vi "PH_Interaction.Super Destroy Me.vi"(0 "i ref out":refnum<vi>) -> ()   [LabVIEW 2014, in "PH_Common.lvlib"]
doc: "This VI forces the super proc asks the super proc to desgtroy the referenced instance."
uses:
  CS_Core/CSSystem/CoreLib/CoreLib.string 2 byte array.vi
  PH_Common.lvlib
  CS_Core/BaseProcess/BaseProcess.lvlib
  CS_Core/CSSystem/CSSystemLib/CSSystemLib.lvlib
  CS_Core/CSSystem/CoreLib/CoreLib.lvlib
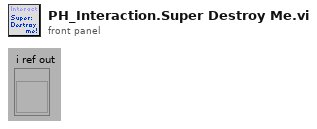
[diagram p1: front panel]
types:
  T1 = typedef "CoreDefs.rawDataType.ctl" = i8[]
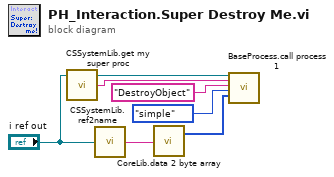
[diagram p0: block diagram]
diagram:
  n1 = call "CSSystemLib.get my super proc.vi"() -> ("name"=w2:string)  [unwired: 1 in]
  n2 = call "CSSystemLib.ref2name.vi"("obj refnum"="i ref out") -> ("name"=w5:string)
  n3 = call-poly "CoreLib.data 2 byte array.vi"("string"=w5) -> ("byteArray out"=w6:T1)  [unwired: 18 in]
  n4 = call "BaseProcess.call process 1.vi"("i ref in"="i ref out", "Object"=w2, "Selector"="DestroyObject", "CallType"=enum16{"simple", "synchronous", "asynchronous"}."simple", "Data"=w6) -> ()  [unwired: 12 in, 3 out]
